vi "Enforce Joint Limits.vi"(8 "error in (no error)":errorcluster, 10 "Joint Command":T1, 11 "Grips Robot in":refnum<class "Grips Robot.lvclass">) -> (0 "error out":errorcluster, 2 "Enforced Command":T1, 3 "Grips Robot out":refnum<class "Grips Robot.lvclass">)   [LabVIEW 2013, in "Grips Robot.lvclass"]
uses:
  Grips Robot.lvclass
  labview_ros/osrf_msgs/JointCommands.ctl
  labview_ros/std_msgs/Header.ctl
  Grips Robot.lvclass/Grips Robot.ctl
  Helpers/Helpers.lvlib
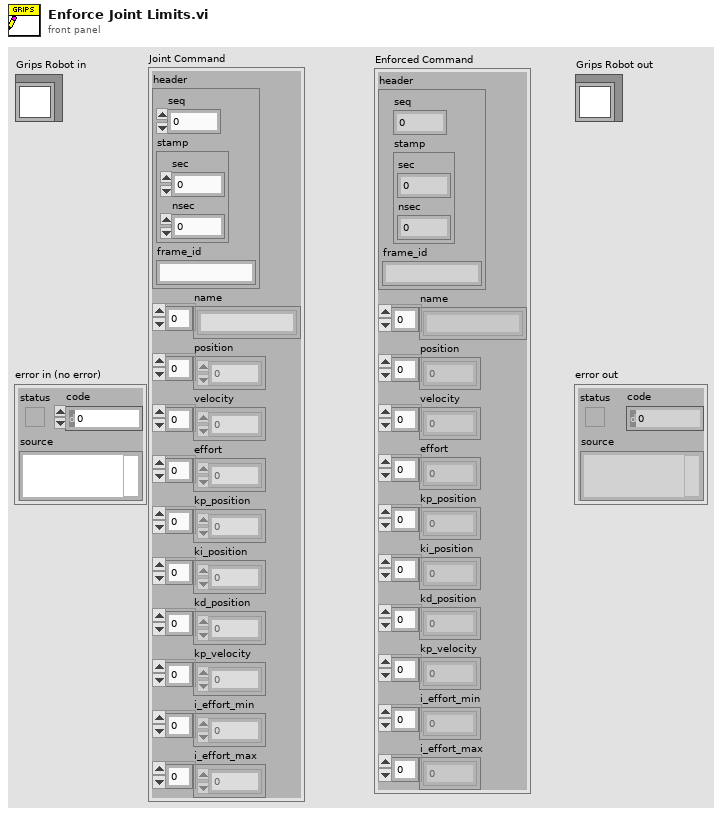
[diagram p1: front panel]
types:
  T1 = typedef "JointCommands.ctl" = cluster{"header":T2, "name":string[], "position":dbl[], "velocity":dbl[], "effort":dbl[], "kp_position":dbl[], "ki_position":dbl[], "kd_position":dbl[], "kp_velocity":dbl[], "i_effort_min":dbl[], "i_effort_max":dbl[]}
  T2 = typedef "Header.ctl" = cluster{"seq":u32, "stamp":cluster{"sec":i32, "nsec":i32}, "frame_id":string}
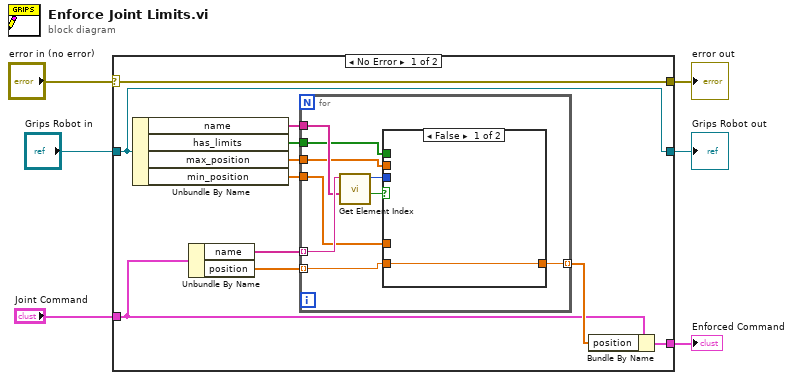
[diagram p0: block diagram]
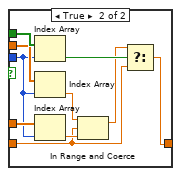
[diagram p2: hidden frame]
diagram:
  n1 = case shown="No Error" "error in (no error)" {
    selector: "error in (no error)" -> [w17 w38]
    tunnel: [w17 w38] -> w5
    tunnel: [w16 w39] -> w3
    tunnel: "Grips Robot in" -> [w16 w39]
    tunnel: "Joint Command" -> [w7 _]
    tunnel: [w10 _] -> w1
    frame No Error {
      n2 = Unbundle By Name(w16) -> ("name"=w15:string[], "has_limits"=w14:bool[], "max_position"=w13:dbl[], "min_position"=w12:dbl[])
      n3 = Unbundle By Name(w7) -> ("name"=w9:string[], "position"=w8:dbl[])
      n4 = for {
        tunnel: w15 -> [w25]
        tunnel: w14 -> [w23]
        tunnel: w13 -> [w22]
        tunnel: w12 -> [w21]
        tunnel: [w18] -> w11 mode=indexing
        tunnel: w9 -> [w26] mode=indexing
        tunnel: w8 -> [w19] mode=indexing
        n5 = call "Get Element Index.vi"("Element"=w26, "List"=w25) -> ("result"=w20:i32, "found?"=w24:bool)  [unwired: 7 in]
        n6 = case shown="False" w24 {
          tunnel: w23 -> [_ w37]
          tunnel: w22 -> [_ w36]
          tunnel: w21 -> [_ w35]
          tunnel: w20 -> [_ w34]
          tunnel: w19 -> [w27 w29]
          tunnel: [w27 w28] -> w18
          frame False {
          }
          frame True {
            n7 = Index Array(array=w37, index=w34) -> (element=w33:bool)
            n8 = Index Array(array=w36, index=w34) -> (element=w31:dbl)
            n9 = Index Array(array=w35, index=w34) -> (element=w32:dbl)
            n10 = In Range and Coerce(upper limit=w31, x=w29, lower limit=w32) -> (coerced(x)=w30:dbl)  [unwired: 1 out]
            n11 = Select(t=w30, s=w33, f=w29) -> (s? t:f=w28:dbl)
          }
        }
      }
      n12 = Bundle By Name(cluster=w7, "position"=w11) -> (w10:T1)
    }
    frame Error {
    }
  }
  "error out" <- w5
  "Grips Robot out" <- w3
  "Enforced Command" <- w1
